vi "Write Command _OC Trim_.vi"(8 "error in (no error)":errorcluster, 10 "Command \"OC Trim\"":string, 11 "LCRControl in":refnum<class "LCRControl.lvclass">) -> (0 "error out":errorcluster, 3 "LCRControl out":refnum<class "LCRControl.lvclass">)   [LabVIEW 2013, in "LCRControl.lvclass"]
uses:
  LCRControl.lvclass
  LCRControl.lvclass/LCRControl.ctl
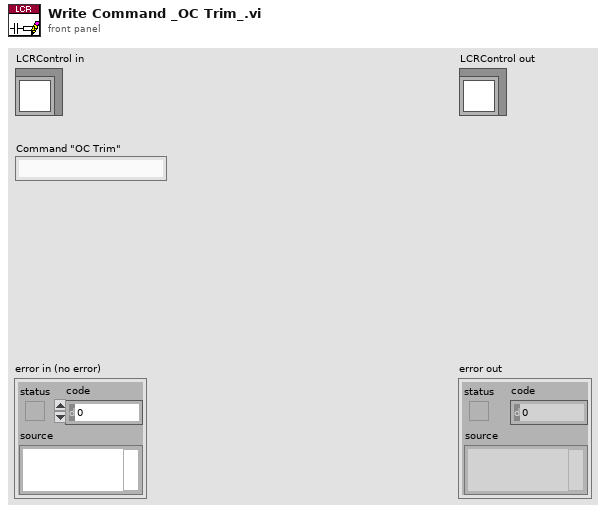
[diagram p1: front panel]
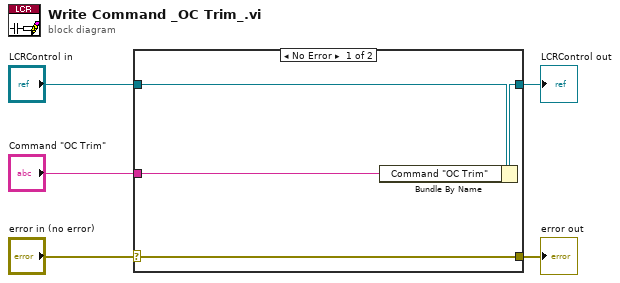
[diagram p0: block diagram]
diagram:
  n1 = case shown="No Error" "error in (no error)" {
    selector: "error in (no error)" -> [w9 w10]
    tunnel: [w9 w10] -> w4
    tunnel: [w7 w11] -> w2
    tunnel: "LCRControl in" -> [w8 w11]
    tunnel: "Command \"OC Trim\"" -> [w6 _]
    frame No Error {
      n2 = Bundle By Name(cluster=w8, "Command \"OC Trim\""=w6) -> (w7:refnum<class "LCRControl.lvclass">)
    }
    frame Error {
    }
  }
  "error out" <- w4
  "LCRControl out" <- w2
